vi "Parse JSON.vi"(8 "error in (no error)":errorcluster, 10 "JSON String":string) -> (0 "error out":errorcluster, 1 "JSON Compatible Type":T1=enum."Unknown", 2 "Root Type":T2=enum."Unknown", 3 "JSON Tree":variant)   [LabVIEW 2010, in "i3-json.lvlib"]
doc: "Use this template to build a VI to use as a subVI."
uses:
  i3-json.lvlib
  JSON Types/JSON Type.ctl
  JSON Types/JSON Compatible Type.ctl
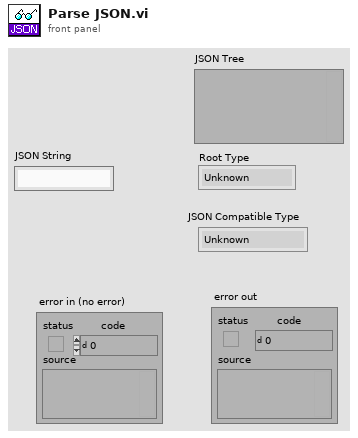
[diagram p1: front panel]
types:
  T1 = typedef "i3-json.lvlib/JSON Compatible Type.ctl" = enum16{"1D Double Array", "1D String Array", "1D Boolean Array", "Unknown"}
  T2 = typedef "i3-json.lvlib/JSON Type.ctl" = enum8{"JSON Compatible", "JSON Array", "JSON Object", "JSON Null", "Double", "String", "Boolean", "Unknown"}
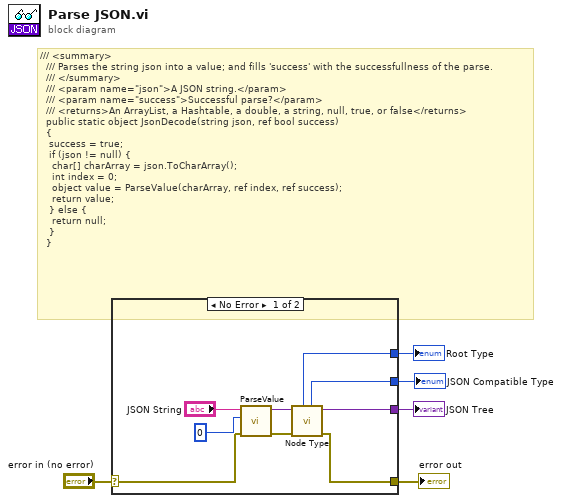
[diagram p0: block diagram]
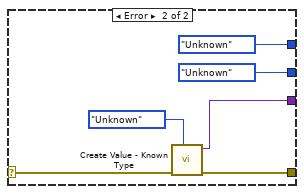
[diagram p2: hidden frame]
diagram:
  # "/// <summary>\n\t\t/// Parses the string json into a value; and fills 'success' with the successfullness of the parse.\n\t\t/// </summary>\n\t\t/// <param name=\"json\">A JSON string.</param>\n\t\t/// <param name=\"success\">Successful parse?</param>\n\t\t/// <returns>An ArrayList, a Hashtable, a double, a string, null, true, or false</returns>\n\t\tpublic static object JsonDecode(string json, ref bool success)\n\t\t{\n\t\t\tsuccess = true;\n\t\t\tif (json != null) {\n\t\t\t\tchar[] charArray = json.ToCharArray();\n\t\t\t\tint index = 0;\n\t\t\t\tobject value = ParseValue(charArray, ref index, ref success);\n\t\t\t\treturn value;\n\t\t\t} else {\n\t\t\t\treturn null;\n\t\t\t}\n\t\t}"
  n1 = case shown="No Error" "error in (no error)" {
    selector: "error in (no error)" -> [w12 w20]
    tunnel: [w11 w19] -> w4
    tunnel: [w8 w18] -> w3
    tunnel: [w7 JSON_Compatible_Type."Unknown" ("JSON Compatible Type")] -> w2
    tunnel: [w6 JSON_Type."Unknown" ("JSON Type")] -> w1
    frame No Error {
      n2 = call "ParseValue.vi"("error in (no error)"=w12, "Index In"=0, "JSON String"="JSON String") -> ("error out"=w10:errorcluster, "JSON Tree"=w9:variant)  [unwired: 6 in, 1 out]
      n3 = call "Node Type.vi"("error in (no error)"=w10, "JSON Tree In"=w9) -> ("error out"=w11:errorcluster, "JSON Tree Passthrough"=w8:variant, "JSON Compatible Type"=w7:T1, "JSON Type"=w6:T2)  [unwired: 5 in, 1 out]
    }
    frame Error {
      n4 = call "Create Value - Known Type.vi"("JSON Type"=JSON_Type."Unknown", "error in (no error)"=w20) -> ("error out"=w19:errorcluster, "JSON Tree"=w18:variant)  [unwired: 8 in]
    }
  }
  "error out" <- w4
  "JSON Tree" <- w3
  "JSON Compatible Type" <- w2
  "Root Type" <- w1
